vi "Color from RGB.vi"(8 "error in (no error)":errorcluster, 10 "Color Box":u32(colorbox), 11 "Color in":refnum<class "Color.lvclass">) -> (0 "error out":errorcluster, 2 "Color":u16, 3 "Color out":refnum<class "Color.lvclass">)   [LabVIEW 2020, in "RPI.SenseHat.Display.lvlib" / "Color.lvclass"]
doc: "Gets Color (RGB565) from LabVIEW Color Box."
uses:
  Color.lvclass
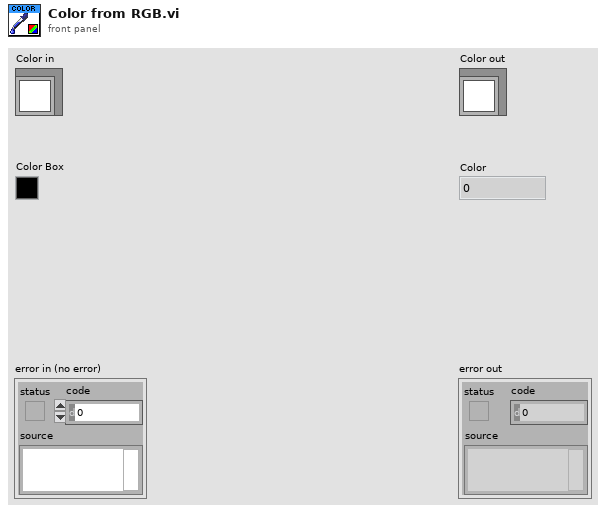
[diagram p1: front panel]
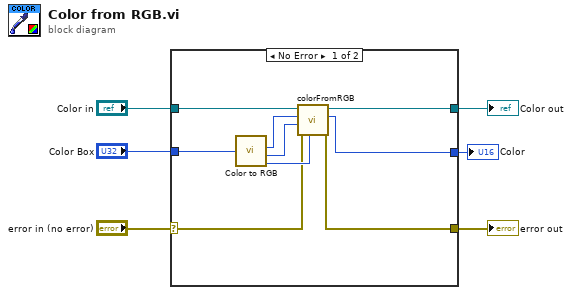
[diagram p0: block diagram]
diagram:
  n1 = case shown="No Error" "error in (no error)" {
    selector: "error in (no error)" -> [w9 w17]
    tunnel: [w8 w17] -> w5
    tunnel: [w14 w16] -> w3
    tunnel: "Color in" -> [w15 w16]
    tunnel: "Color Box" -> [w10 _]
    tunnel: [w7 _] -> w1
    frame No Error {
      n2 = call <vilib>:"Color to RGB.vi"("Color"=w10) -> ("R"=w13:u8, "G"=w12:u8, "B"=w11:u8)  [unwired: 1 out]
      n3 = call "colorFromRGB.vi"("Blue"=w11, "error in (no error)"=w9, "Green"=w12, "Red"=w13, "Color in"=w15) -> ("error out"=w8:errorcluster, "Color"=w7:u16, "Color out"=w14:refnum<class "Color.lvclass">)  [unwired: 4 in]
    }
    frame Error {
    }
  }
  "error out" <- w5
  "Color out" <- w3
  "Color" <- w1
